vi "Cross Correlation Peak Search.vi"(5 "consecutive samples over threshold":u8, 7 "square of cross correlation magnitude threshold":fxp<+,18,1> format="%#_18g", 9 "input valid":bool, 10 "normalized cross correlation":T1) -> (1 "peak found":bool, 2 "peak index":u16)   [LabVIEW 2020]
uses:
  <vilib>/rvi/FXPMathLib/FxpInterpret/XNode/nifxpmath_Interpret.xnode
types:
  T1 = cluster{"Real":fxp<+/-,18,1>, "Imag":fxp<+/-,18,1>}
  T2 = cluster{"Real":fxp<+/-,25,25>, "Imag":fxp<+/-,25,25>}
  T3 = cluster{"Real":fxp<+/-,18,18>, "Imag":fxp<+/-,18,18>}
  T4 = cluster{"Real":fxp<+/-,48,48>, "Imag":fxp<+/-,48,48>}
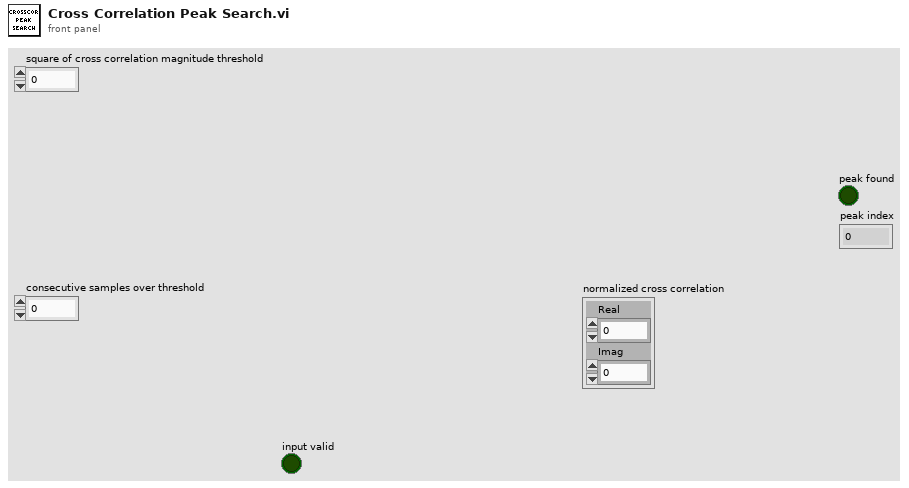
[diagram p1: front panel]
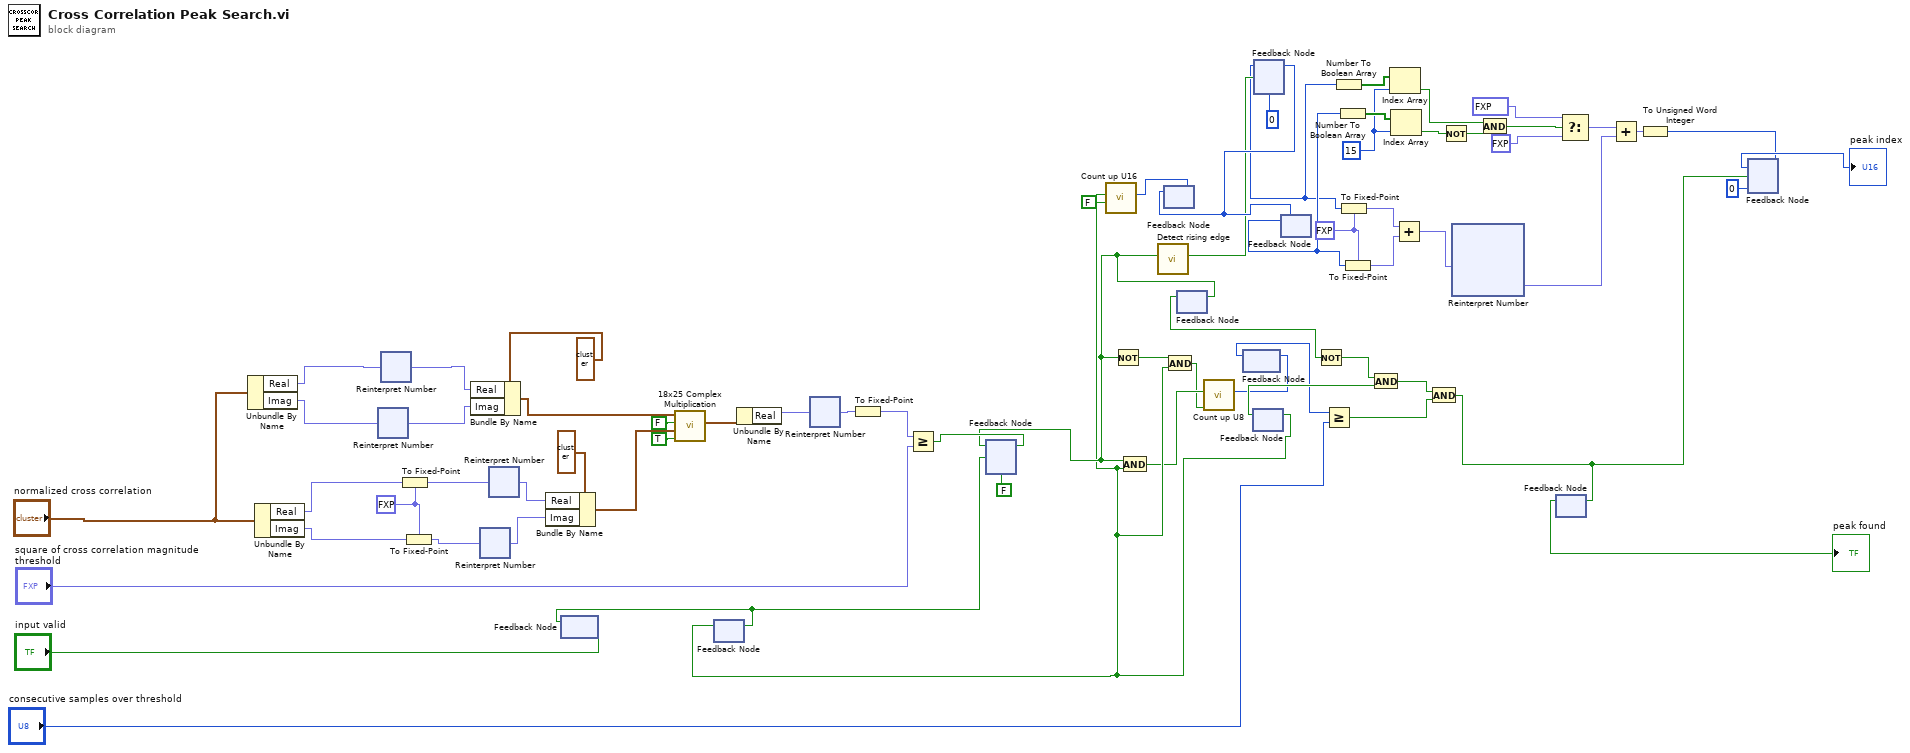
[diagram p0: block diagram]
diagram:
  w7 = 15 ("index")
  w20 = fxp<+,16,16> 0.0 ("fixed-point type")
  w68 = fxp<+/-,25,8> 0.0 ("fixed-point type")
  n1 = Unbundle By Name("normalized cross correlation") -> ("Real"=w58:fxp<+/-,18,1>, "Imag"=w56:fxp<+/-,18,1>)
  n2 = Unbundle By Name("normalized cross correlation") -> ("Real"=w67:fxp<+/-,18,1>, "Imag"=w66:fxp<+/-,18,1>)
  n3 = xnode "Reinterpret Number"("x"=w56) -> ("y"=w55:fxp<+/-,18,18>)
  n4 = xnode "Reinterpret Number"("x"=w58) -> ("y"=w57:fxp<+/-,18,18>)
  n5 = To Fixed-Point(fixed-point type=w68, number=w67) -> (fixed-point=w54:fxp<+/-,25,8>)
  n6 = To Fixed-Point(fixed-point type=w68, number=w66) -> (fixed-point=w52:fxp<+/-,25,8>)
  n7 = Bundle By Name(cluster=T3 {"Real"=0.0, "Imag"=0.0} ("A"), "Real"=w57, "Imag"=w55) -> (w63:T3)
  n8 = xnode "Reinterpret Number"("x"=w52) -> ("y"=w51:fxp<+/-,25,25>)
  n9 = xnode "Reinterpret Number"("x"=w54) -> ("y"=w53:fxp<+/-,25,25>)
  n10 = Bundle By Name(cluster=T2 {"Real"=0.0, "Imag"=0.0} ("B"), "Real"=w53, "Imag"=w51) -> (w59:T2)
  n11 = feedback-in #1("input valid") -> ()
  n12 = feedback #1() -> (w42:bool)  [unwired: 1 in]
  n13 = call "18x25 Complex Multiplication.vi"("conjugate B"=TRUE, "B"=w59, "conjugate A"=FALSE, "A"=w63) -> ("product"=w50:T4)  [unwired: 7 in]
  n14 = feedback #2() -> (w33:bool)  [unwired: 1 in]
  n15 = feedback-in #2(w42) -> ()
  n16 = Unbundle By Name(w50) -> ("Real"=w49:fxp<+/-,48,48>)
  n17 = xnode "Reinterpret Number"("x"=w49) -> ("y"=w48:fxp<+/-,48,14>)
  n18 = To Fixed-Point(number=w48) -> (fixed-point=w47:fxp<+/-,48,14>)  [unwired: 1 in]
  n19 = Greater Or Equal?(x=w47, y="square of cross correlation magnitude threshold") -> (x >= y?=w45:bool)
  n20 = feedback-in #3(w45, w42) -> ()
  n21 = feedback #3(FALSE) -> (w36:bool)
  n22 = call "Count up U16.vi"("reset"=FALSE, "increment"=w33) -> ("count out"=w39:u16)  [unwired: 9 in]
  n23 = Not(x=w36) -> (.not. x?=w41:bool)
  n24 = And(x=w36, y=w33) -> (x .and. y?=w28:bool)
  n25 = call "Detect rising edge.vi"("signal"=w36) -> ("edge detected"=w37:bool)  [unwired: 10 in]
  n26 = feedback #4() -> (w38:u16)  [unwired: 1 in]
  n27 = feedback-in #4(w39) -> ()
  n28 = And(x=w41, y=w33) -> (x .and. y?=w27:bool)
  n29 = feedback #5() -> (w35:bool)  [unwired: 1 in]
  n30 = feedback-in #5(w36) -> ()
  n31 = call "Count up U8.vi"("reset"=w27, "increment"=w28) -> ("count out"=w25:u8)  [unwired: 9 in]
  n32 = feedback #6() -> (w26:u8)  [unwired: 1 in]
  n33 = feedback-in #6(w25) -> ()
  n34 = feedback #7() -> (w32:bool)  [unwired: 1 in]
  n35 = feedback-in #7(w33) -> ()
  n36 = feedback #8(u16 0 ("count out")) -> (w10:u16)
  n37 = feedback-in #8(w38, w37) -> ()
  n38 = feedback #9() -> (w11:u16)  [unwired: 1 in]
  n39 = feedback-in #9(w38) -> ()
  n40 = Not(x=w35) -> (.not. x?=w34:bool)
  n41 = Greater Or Equal?(x=w26, y="consecutive samples over threshold") -> (x >= y?=w30:bool)
  n42 = Number To Boolean Array(number=w10) -> (Boolean array=w9:bool[])
  n43 = Number To Boolean Array(number=w11) -> (Boolean array=w8:bool[])
  n44 = To Fixed-Point(fixed-point type=w20, number=w10) -> (fixed-point=w19:fxp<+,16,16>)
  n45 = To Fixed-Point(fixed-point type=w20, number=w11) -> (fixed-point=w18:fxp<+,16,16>)
  n46 = And(x=w34, y=w32) -> (x .and. y?=w31:bool)
  n47 = Index Array(array=w9, index=w7) -> (element=w3:bool)
  n48 = Index Array(array=w8, index=w7) -> (element=w5:bool)
  n49 = Add(x=w19, y=w18) -> (x+y=w17:fxp<+,17,17>)
  n50 = And(x=w31, y=w30) -> (x .and. y?=w23:bool)
  n51 = Not(x=w5) -> (.not. x?=w4:bool)
  n52 = xnode "Reinterpret Number"("x"=w17) -> ("y"=w15:fxp<+,17,16>)
  n53 = And(x=w3, y=w4) -> (x .and. y?=w6:bool)
  n54 = feedback #10() -> (→"peak found":bool)  [unwired: 1 in]
  n55 = feedback-in #10(w23) -> ()
  n56 = Select(t=fxp<+,17,16> 32768.0 ("y"), s=w6, f=fxp<+,17,16> 0.0 ("y")) -> (s? t:f=w14:fxp<+,17,16>)
  n57 = Add(x=w14, y=w15) -> (x+y=w16:fxp<+,16,16>)
  n58 = To Unsigned Word Integer(number=w16) -> (unsigned 16bit integer=w21:u16)
  n59 = feedback #11(u16 0) -> (→"peak index":u16)
  n60 = feedback-in #11(w21, w23) -> ()
